vi "VCS Stop Homing.vi"(8 "error in (no error)":errorcluster, 11 "axis in":cluster{"keyHandle":u32, "nodeId":u16}={"keyHandle"=0, "nodeId"=1}) -> (0 "error out":errorcluster, 3 "axis out":cluster{"keyHandle":u32, "nodeId":u16}={"keyHandle"=0, "nodeId"=1})   [LabVIEW 2019]
doc: "<B>VCS Stop Homing</B> interrupts homing."
uses:
  Resources/EposCmd.dll
  Resources/EposCmd64.dll
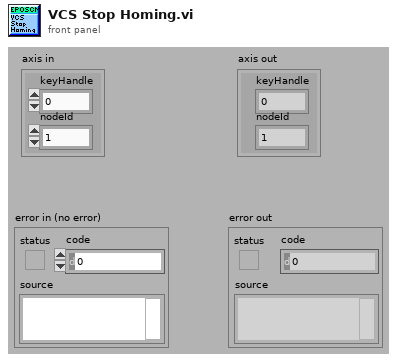
[diagram p1: front panel]
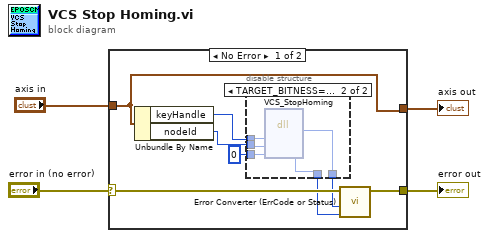
[diagram p0: block diagram]
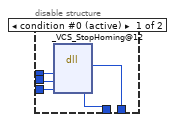
[diagram p2: hidden frame]
diagram:
  n1 = case shown="No Error" "error in (no error)" {
    selector: "error in (no error)" -> [w12 w24]
    tunnel: [w11 w24] -> w3
    tunnel: "axis in" -> [w7 w23]
    tunnel: [w7 w23] -> w1
    frame No Error {
      n2 = Unbundle By Name(w7) -> ("keyHandle"=w9:u32, "nodeId"=w8:u16)
      n3 = disable-structure shown="TARGET_BITNESS==64" {
        disable-tunnel: [w17 w22] -> w10
        disable-tunnel: w9 -> [w16 w21]
        disable-tunnel: w8 -> [w15 w20]
        disable-tunnel: [w14 w19] -> w6
        disable-tunnel: u32 0 ("pErrorCode") -> [w13 w18]
        frame condition #0 (active) {
          n4 = dll-call lib="C:/Projeto em LabVIEW/EPOS-LabVIEW-Instrument-Driver-En/LabVIEW/maxon EPOS/Resources/EposCmd.*" fn="_VCS_StopHoming@12"("KeyHandle"=w16, "NodeId"=w15, "pErrorCode"=w13) -> (w14:i32, "pErrorCode"=w17:u32)  [unwired: 5 in, 2 out]
        }
        frame condition #1 {
          n5 = dll-call lib="C:/setup/Resources/EposCmd64.*" fn="VCS_StopHoming" ("EposCmd.dll:_VCS_StopHoming@12")("KeyHandle"=w21, "NodeId"=w20, "pErrorCode"=w18) -> ("Rückgabetyp"=w19:i32, "pErrorCode"=w22:u32)  [unwired: 5 in, 2 out]
        }
      }
      n6 = call "Error Converter (ErrCode or Status).vi"("error code"=w10, "return type"=w6, "error in (no error)"=w12) -> ("error out"=w11:errorcluster)  [unwired: 7 in]
    }
    frame Error {
    }
  }
  "error out" <- w3
  "axis out" <- w1
